vi "保存数据基层VI.vi"(0 "输入完整路径(.csv)":path, 1 "第二表头":string[](array[string]), 5 "表头":string[](array[string]), 7 "文件行数":dbl, 9 "数据":string[](array[string]), 11 "error in (no error)":errorcluster caption="错误输入（无错误）", 12 "文件行数大小":dbl=32000.0) -> (4 "输出完整路径(.csv)":path, 14 "error out":errorcluster, 15 "文件行数输出":dbl)   [LabVIEW 2013]
uses:
  <vilib>/Utility/file.llb/Write To Spreadsheet File (string).vi
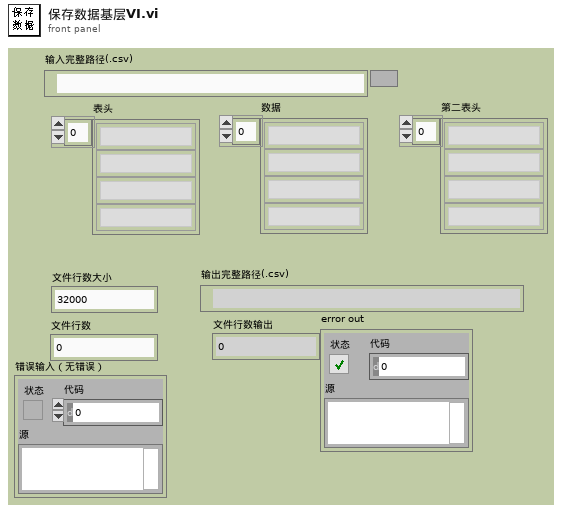
[diagram p1: front panel]
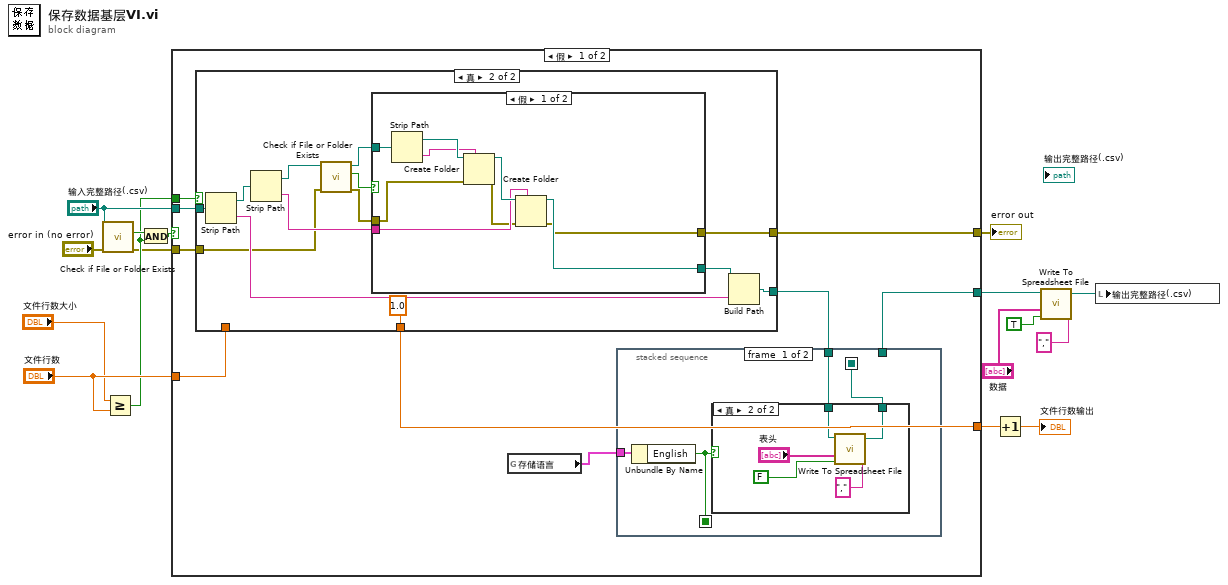
[diagram p0: block diagram]
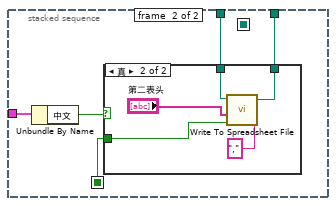
[diagram p3: hidden frame]
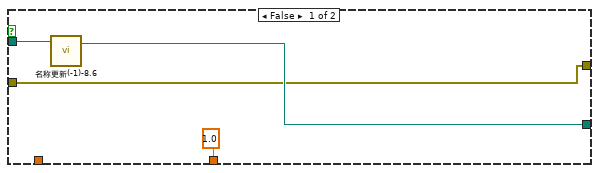
[diagram p5: hidden frame]
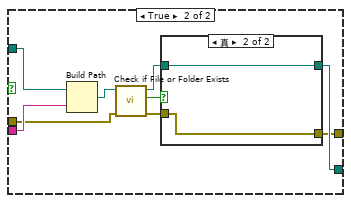
[diagram p6: hidden frame]
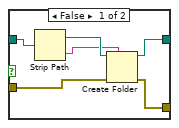
[diagram p7: hidden frame]
diagram:
  n1 = call <vilib>:"Check if File or Folder Exists.vi"("error in (no error)"="error in (no error)", "path"="输入完整路径(.csv)") -> ("error out"=w3:errorcluster, "file or folder exists?"=w7:bool)  [unwired: 8 out]
  n2 = Greater Or Equal?(x="文件行数大小", y="文件行数") -> (x >= y?=w6:bool)
  n3 = And(x=w7, y=w6) -> (x .and. y?=w11:bool)
  n4 = case shown="假" w11 {
    tunnel: "输入完整路径(.csv)" -> [w25 w92]
    tunnel: [w23 w92] -> w15
    tunnel: "文件行数" -> [w22 w91]
    tunnel: [w21 w91] -> w10
    tunnel: w6 -> [w20 _]
    tunnel: w3 -> [w18 w90]
    tunnel: [w17 w90] -> w1
    frame False {
      n5 = case shown="真" w20 {
        tunnel: w25 -> [w50 w56]
        tunnel: [w49 w55] -> w24
        tunnel: w22 -> [_ _]
        tunnel: [1.0 ("文件行数") 1.0 ("文件行数")] -> w21
        tunnel: w18 -> [w47 w52]
        tunnel: [w47 w51] -> w17
        frame False {
          n6 = call "名称更新(-1)-8.6.vi"("输入"=w50) -> ("输出"=w49:path)  [unwired: 2 out]
        }
        frame True {
          n7 = Strip Path(path=w56) -> (stripped path=w63:path, name=w58:string)
          n8 = Strip Path(path=w63) -> (stripped path=w62:path, name=w61:string)
          n9 = call <vilib>:"Check if File or Folder Exists.vi"("error in (no error)"=w52, "path"=w62) -> ("error out"=w53:errorcluster, "file or folder exists?"=w57:bool, "dup path"=w60:path)  [unwired: 7 out]
          n10 = case shown="假" w57 {
            tunnel: w61 -> [w67 w77]
            tunnel: w60 -> [w72 w78]
            tunnel: [w71 w76] -> w59
            tunnel: w53 -> [w65 w75]
            tunnel: [w66 w73] -> w51
            frame False {
              n11 = Strip Path(path=w72) -> (stripped path=w70:path, name=w69:string)
              n12 = Create Folder(prompt (Create Folder)=w69, path (use dialog)=w70, error in=w65) -> (created path=w68:path, error out=w64:errorcluster)  [unwired: 1 out]
              n13 = Create Folder(prompt (Create Folder)=w67, path (use dialog)=w68, error in=w64) -> (created path=w71:path, error out=w66:errorcluster)  [unwired: 1 out]
            }
            frame True {
              n14 = Build Path(base path=w78, name or relative path=w77) -> (appended path=w80:path)
              n15 = call <vilib>:"Check if File or Folder Exists.vi"("error in (no error)"=w75, "path"=w80) -> ("error out"=w74:errorcluster, "file or folder exists?"=w81:bool, "dup path"=w79:path)  [unwired: 7 out]
              n16 = case shown="真" w81 {
                tunnel: w79 -> [w87 w89]
                tunnel: [w84 w89] -> w76
                tunnel: w74 -> [w83 w88]
                tunnel: [w82 w88] -> w73
                frame False {
                  n17 = Strip Path(path=w87) -> (stripped path=w86:path, name=w85:string)
                  n18 = Create Folder(prompt (Create Folder)=w85, path (use dialog)=w86, error in=w83) -> (created path=w84:path, error out=w82:errorcluster)  [unwired: 1 out]
                }
                frame True {
                }
              }
            }
          }
          n19 = Build Path(base path=w59, name or relative path=w58) -> (appended path=w55:path)
        }
      }
      n20 = global read "EV05全局变量1.vi" "存储语言"() -> (w19:cluster{"English":bool, "中文":bool})
      n21 = stacked-sequence {
        seq-local: [w26 _] -> [_ _]
        seq-local: [w27 _] -> [_ w37]
        tunnel: w24 -> [w29 w40]
        tunnel: [_ w36] -> w23
        tunnel: w19 -> [w28 w39]
        frame #0 {
          n22 = Unbundle By Name(w28) -> ("English"=w27:bool)
          n23 = case shown="真" w27 {
            tunnel: w29 -> [w30 w35]
            tunnel: [w30 w31] -> w26
            frame False {
            }
            frame True {
              n24 = call-poly <vilib>:"Write To Spreadsheet File.vi"("delimiter (\\t)"="," ("delimiter (\\t)"), "append to file? (new file:F)"=FALSE, "1D data"="表头", "file path (dialog if empty)"=w35) -> ("new file path (Not A Path if cancelled)"=w31:path)  [unwired: 3 in, 1 out]
            }
          }
        }
        frame #1 {
          n25 = Unbundle By Name(w39) -> ("中文"=w38:bool)
          n26 = case shown="真" w38 {
            tunnel: w40 -> [w41 w46]
            tunnel: [w41 w44] -> w36
            tunnel: w37 -> [_ w42]
            frame False {
            }
            frame True {
              n27 = call-poly <vilib>:"Write To Spreadsheet File.vi"("delimiter (\\t)"="," ("delimiter (\\t)"), "append to file? (new file:F)"=w42, "1D data"="第二表头", "file path (dialog if empty)"=w46) -> ("new file path (Not A Path if cancelled)"=w44:path)  [unwired: 3 in, 1 out]
            }
          }
        }
      }
    }
    frame True {
    }
  }
  "error out" <- w1
  n28 = Increment(x=w10) -> (x+1=→"文件行数输出":dbl)
  n29 = call-poly <vilib>:"Write To Spreadsheet File.vi"("delimiter (\\t)"="," ("delimiter (\\t)"), "append to file? (new file:F)"=TRUE, "1D data"="数据", "file path (dialog if empty)"=w15) -> ("new file path (Not A Path if cancelled)"=w4:path)  [unwired: 3 in, 1 out]
  n30 = local write "输出完整路径(.csv)"(w4) -> ()
